vi "Save PNG Image of Front Panel.vi"(8 "error in (no error)":errorcluster, 10 "VI Path":path, 11 "File Path In":path) -> (0 "error out":errorcluster, 3 "File Path Out":path)   [LabVIEW 2012]
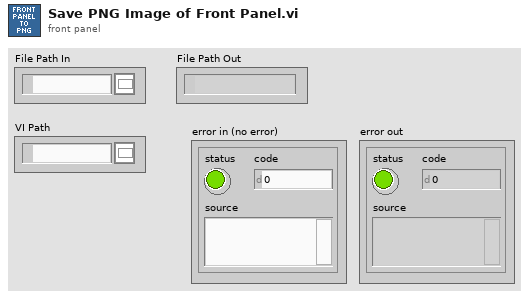
[diagram p1: front panel]
types:
  T1 = typedef "imagedata.ctl" = cluster{"image type":i32, "image depth":i32, "image":u8[], "mask":u8[], "colors":u32[], "Rectangle":cluster{"left":i16, "top":i16, "right":i16, "bottom":i16}}
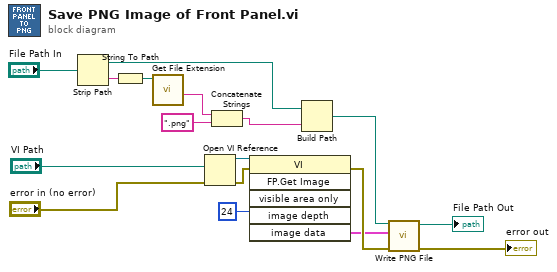
[diagram p0: block diagram]
diagram:
  n1 = Strip Path(path="File Path In") -> (stripped path=w2:path, name=w7:string)
  n2 = String To Path(string=w7) -> (path=w6:path)
  n3 = call <vilib>:"Get File Extension.vi"("file"=w6) -> ("filename without extension"=w5:string)  [unwired: 7 in, 3 out]
  n4 = Open VI Reference(vi path="VI Path", error in (no error)="error in (no error)") -> (vi reference=w10:refnum<vi>, error out=w14:errorcluster)  [unwired: 4 in]
  n5 = Concatenate Strings(w5, ".png" ("string")) -> (w3:string)
  n6 = invoke class="VI" method="FP.Get Image"(reference=w10, error in=w14, "image depth"=24 ("Image Depth")) -> (error out=w15:errorcluster, "image data"=w11:T1)  [unwired: 3 in, 4 out]
  n7 = Build Path(base path=w2, name or relative path=w3) -> (appended path=w1:path)
  n8 = call <vilib>:"Write PNG File.vi"("error in (no error)"=w15, "image data"=w11, "path to PNG file"=w1) -> ("error out"=→"error out":errorcluster, "path"=→"File Path Out":path)  [unwired: 7 in]
